vi "Teleop.vi"(10 "Match Info":T1={"Autonomous Elapsed Seconds"=0.0, "TeleOp Elapsed Seconds"=0.0, "Disabled Elapsed Seconds"=0.0, "Visited Autonomous"=FALSE, "Visited TeleOp"=FALSE, "Visited Disabled"=FALSE, "Autonomous Settings"={"Autonomous Style"=enum."Independent", "VI Refnum"=refnum}}, 11 "Call Context":T2) -> ()   [LabVIEW 2015]
doc: "This VI is called for each TeleOp packet received from the DS where the robot is not disabled. It is often used to read from the joysticks and update I/O or to update setpoints for timed control loops. It should complete and return within 20 milliseconds or it may miss DS packets."
uses:
  <vilib>/Rock Robotics/WPI/DriverStation/WPI_DriverStationDerivedRobotMode.ctl
  <vilib>/Rock Robotics/WPI/DriverStation/WPI_DriverStationMatch Info.ctl
  <vilib>/Rock Robotics/Network Tables/NT Read Boolean.vi
  <vilib>/Rock Robotics/Network Tables/NT Read Number.vi
  <vilib>/Rock Robotics/WPI/Utilities/WPI_GetSetVariantRefNum.vi
  Robot Global Data.vi
  <vilib>/Rock Robotics/Network Tables/SD Write Boolean.vi
  <vilib>/Rock Robotics/Network Tables/SD Write Number.vi
  navX Library v2/navX Library v2.lvlib
panel:
  in  "Speed":dbl
  out "Sample Slider 0":dbl(slide) scale=0.0..5.0
  out "Sample Boolean 1":bool
  out "Sample Boolean 0":bool
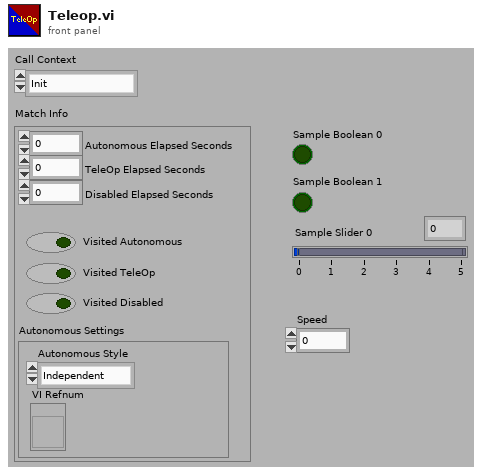
[diagram p1: front panel]
types:
  T1 = typedef "WPI_DriverStationMatch Info.ctl" = cluster{"Autonomous Elapsed Seconds":dbl, "TeleOp Elapsed Seconds":dbl, "Disabled Elapsed Seconds":dbl, "Visited Autonomous":bool, "Visited TeleOp":bool, "Visited Disabled":bool, "Autonomous Settings":cluster{"Autonomous Style":enum16{"Iterative", "Independent"}, "VI Refnum":refnum<vi>}}
  T2 = typedef "WPI_DriverStationDerivedRobotMode.ctl" = enum16{"Init", "Execute", "Stop"}
  T3 = typedef "navX Library v2.lvlib/Z900_navX_DeviceTypeDef.ctl" = cluster{"Interface":cluster{"Protocol":T4, "Update Rate (4Hz-60Hz)":u8, "navX Open TypeDef":variant}, "Notify Packet":refnum<notifier>, "Loop VI Refnum":refnum<vi>, "Ready to Close Occurrence Refnum":refnum<k4>}
  T4 = typedef "navX Library v2.lvlib/Z900_navX_ProtocolTypeDef.ctl" = enum16{"SERIAL", "I2C", "SPI"}
  T5 = cluster{"LinearAcceleration X":dbl, "LinearAcceleration Y":dbl, "LinearAcceleration Z":dbl}
  T6 = cluster{"Velocity X":dbl, "Velocity Y":dbl, "Velocity Z":dbl, "Displacement X":dbl, "Displacement Y":dbl, "Displacement Z":dbl}
  T7 = cluster{"Quat W":dbl, "Quat X":dbl, "Quat Y":dbl, "Quat Z":dbl}
  T8 = cluster{"Yaw":dbl, "Roll":dbl, "Pitch":dbl, "Heading":dbl, "Fused Heading":dbl}
  T9 = typedef "WPI_JoystickDevRef.ctl" = cluster{"Device":T10}
  T10 = typedef "WPI_JoystickDeviceEnum.ctl" = enum16{"USB 0", "USB 1", "USB 2", "USB 3", "USB 4", "USB 5"}
  T11 = cluster{"Axes[0]":dbl, "Axes[1]":dbl, "Axes[2]":dbl, "Axes[3]":dbl, "Axes[4]":dbl, "Axes[5]":dbl, "Axes[6]":dbl, "Axes[7]":dbl, "Axes[8]":dbl}
  T12 = cluster{"Buttons[0]":bool, "Buttons[1]":bool, "Buttons[2]":bool, "Buttons[3]":bool, "Buttons[4]":bool, "Buttons[5]":bool, "Buttons[6]":bool, "Buttons[7]":bool, "Buttons[8]":bool}
  T13 = typedef "WPI_EncoderDevRef.ctl" = cluster{"DevStatus":errorcluster, "EncoderIndex":T14, "CounterIndex":T15, "DistancePerCount":dbl, "Decoding Type":T16}
  T14 = typedef "FPGA_EncoderIdx.ctl" = enum8{"Enc 0", "Enc 1", "Enc 2", "Enc 3", "Enc 4", "Enc 5", "Enc 6", "Enc 7", "Invalid"}
  T15 = typedef "FPGA_CounterCtrSystemIndex.ctl" = enum8{"Ctr 0", "Ctr 1", "Ctr 2", "Ctr 3", "Ctr 4", "Ctr 5", "Ctr 6", "Ctr 7", "Invalid"}
  T16 = typedef "WPI_EncoderType.ctl" = enum16{"1x", "2x", "4x"}
  T17 = typedef "WPI_RobotDriveDevRef.ctl" = cluster{"DevStatus":errorcluster, "Motors[]":T18[], "Square Inputs":bool, "Max Output":dbl}
  T18 = typedef "WPI_MotorControlDeviceRef.ctl" = cluster{"DeviceStatus":errorcluster, "Type":T19, "PWM":cluster{"PWM Channel":T20, "DeadBand":T21}, "CAN":cluster{"Device Number":u8, "Control Mode":T22, "Semaphore":T23, "Max Vout":dbl, "TalonSRX Control Mode":T24}, "Invert":bool}
  T19 = typedef "WPI_MotorControlType.ctl" = enum16{"PWM", "CAN", "CANTalonSRX"}
  T20 = typedef "FPGA_DIOPWMChannel.ctl" = enum8{"PWM 0", "PWM 1", "PWM 2", "PWM 3", "PWM 4", "PWM 5", "PWM 6", "PWM 7", "PWM 8", "PWM 9", "PWM MXP 0", "PWM MXP 1", "PWM MXP 2", "PWM MXP 3", "PWM MXP 4", "PWM MXP 5", "PWM MXP 6", "PWM MXP 7", "PWM MXP 8", "PWM MXP 9", "Invalid"}
  T21 = typedef "WPI_PWMDeadband.ctl" = cluster{"Name":string, "maxPositivePwm":i32, "minPositivePwm":i32, "centerPwm":i32, "maxNegativePwm":i32, "minNegativePwm":i32, "angularRange":u16}
  T22 = typedef "WPI_CANJaguar_ControlMode.ctl" = enum8{"Percent VBus", "Current", "Speed", "Position", "Voltage"}
  T23 = typedef "Semaphore RefNum" = refnum<k1>
  T24 = typedef "WPI_CANTalonSRX_APIControlMode.ctl" = enum8{"Percent VBus", "Speed", "Position", "Slave", "Unchanged / Invalid", "Voltage Compensation", "Current", "Motion Profile"}
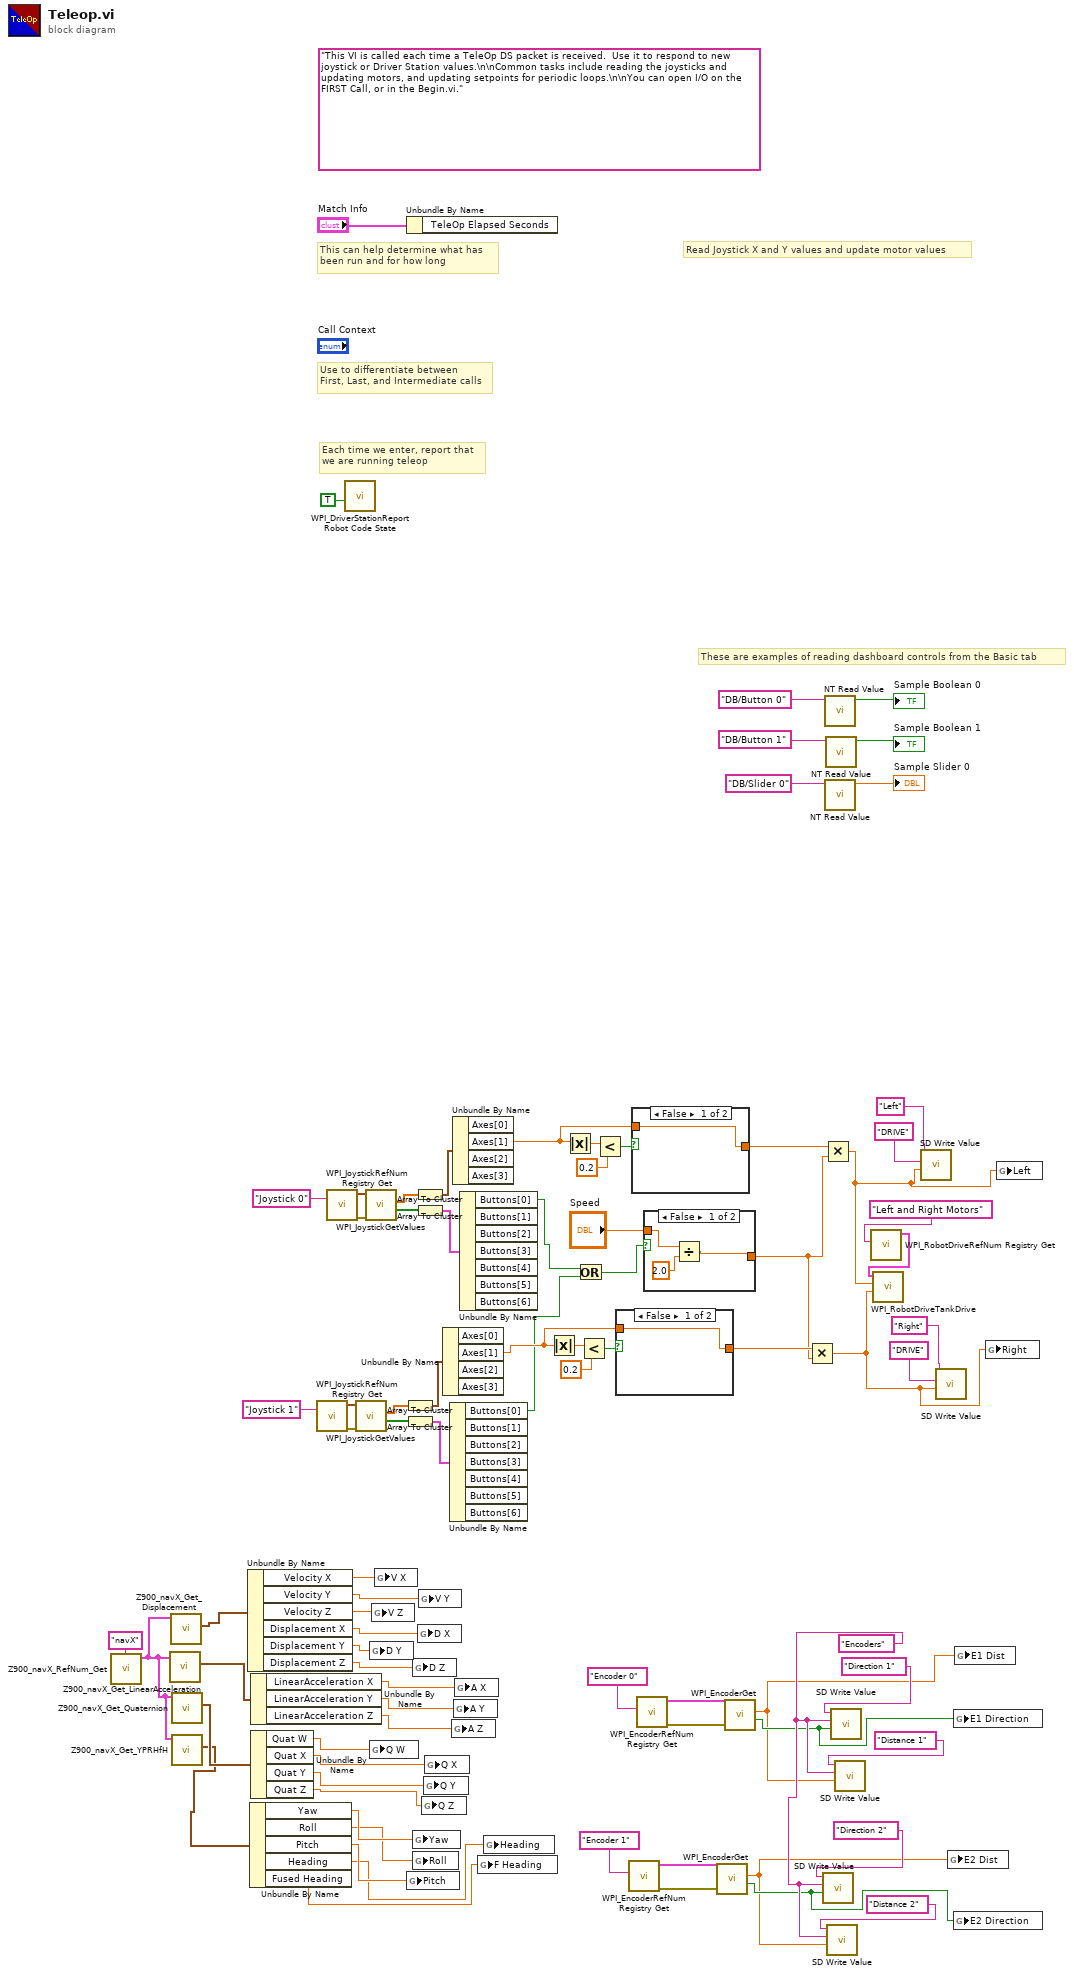
[diagram p0: block diagram]
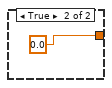
[diagram p3: hidden frame]
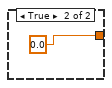
[diagram p4: hidden frame]
diagram:
  w33 = "Encoders"
  (unwired) "This VI is called each time a TeleOp DS packet is received.  Use it to respond to new joystick or Driver Station values.\n\nCommon tasks include reading the joysticks and updating motors, and updating setpoints for periodic loops.\n\nYou can open I/O on the FIRST Call, or in the Begin.vi."
  # "These are examples of reading dashboard controls from the Basic tab"
  # "Each time we enter, report that\nwe are running teleop"
  # "Use to differentiate between\nFirst, Last, and Intermediate calls"
  # "This can help determine what has\nbeen run and for how long"
  # "Read Joystick X and Y values and update motor values"
  n1 = call "Z900_navX_RefNum_Get.vi"("refnum name"="navX") -> ("navX Device"=w24:T3)  [unwired: 9 in, 1 out]
  n2 = call "Z900_navX_Get_LinearAcceleration.vi"("navX Device"=w24) -> ("Linear Acceleration"=w22:T5)  [unwired: 7 in, 3 out]
  n3 = call "Z900_navX_Get_Displacement.vi"("navX Device"=w24) -> ("Displacement"=w23:T6)  [unwired: 7 in, 3 out]
  n4 = call "Z900_navX_Get_Quaternion.vi"("navX Device"=w24) -> ("Quaternion"=w21:T7)  [unwired: 7 in, 3 out]
  n5 = call "Z900_navX_Get_YPRHfH.vi"("navX Device"=w24) -> ("YRPHfH"=w20:T8)  [unwired: 7 in, 3 out]
  n6 = Unbundle By Name(w23) -> ("Velocity X"=w18:dbl, "Velocity Y"=w17:dbl, "Velocity Z"=w16:dbl, "Displacement X"=w15:dbl, "Displacement Y"=w14:dbl, "Displacement Z"=w13:dbl)
  n7 = Unbundle By Name(w20) -> ("Yaw"=w6:dbl, "Roll"=w5:dbl, "Pitch"=w4:dbl, "Heading"=w2:dbl, "Fused Heading"=w1:dbl)
  n8 = Unbundle By Name(w22) -> ("LinearAcceleration X"=w12:dbl, "LinearAcceleration Y"=w11:dbl, "LinearAcceleration Z"=w10:dbl)
  n9 = Unbundle By Name(w21) -> ("Quat W"=w3:dbl, "Quat X"=w9:dbl, "Quat Y"=w8:dbl, "Quat Z"=w7:dbl)
  n10 = call <vilib>:"WPI_JoystickRefNum Registry Get.vi"("refnum name"="Joystick 1") -> ("error out"=w68:errorcluster, "JoystickDevRef"=w25:T9)  [unwired: 9 in]
  n11 = call <vilib>:"WPI_JoystickRefNum Registry Get.vi"("refnum name"="Joystick 0") -> ("error out"=w75:errorcluster, "JoystickDevRef"=w74:T9)  [unwired: 9 in]
  n12 = call <vilib>:"WPI_DriverStationReport Robot Code State.vi"("TeleOp"=TRUE ("Autonomous")) -> ()  [unwired: 10 in, 1 out]
  n13 = call <vilib>:"WPI_JoystickGetValues.vi"("error in (no error)"=w68, "JoystickDevRef"=w25) -> ("Buttons"=w66:bool[], "Axes"=w67:dbl[])  [unwired: 5 in, 3 out]
  n14 = call <vilib>:"WPI_JoystickGetValues.vi"("error in (no error)"=w75, "JoystickDevRef"=w74) -> ("Buttons"=w72:bool[], "Axes"=w73:dbl[])  [unwired: 5 in, 3 out]
  n15 = global write "Robot Global Data.vi" "D Y"(w14) -> ()
  n16 = global write "Robot Global Data.vi" "Q W"(w3) -> ()
  n17 = global write "Robot Global Data.vi" "V Z"(w16) -> ()
  n18 = global write "Robot Global Data.vi" "V X"(w18) -> ()
  n19 = Array To Cluster(array=w67) -> (cluster=w65:T11)
  n20 = Array To Cluster(array=w66) -> (cluster=w64:T12)
  n21 = Unbundle By Name("Match Info") -> ()  [unwired: 1 out]
  n22 = global write "Robot Global Data.vi" "Pitch"(w4) -> ()
  n23 = global write "Robot Global Data.vi" "D Z"(w13) -> ()
  n24 = global write "Robot Global Data.vi" "Yaw"(w6) -> ()
  n25 = global write "Robot Global Data.vi" "Roll"(w5) -> ()
  n26 = Array To Cluster(array=w73) -> (cluster=w71:T11)
  n27 = Array To Cluster(array=w72) -> (cluster=w70:T12)
  n28 = global write "Robot Global Data.vi" "D X"(w15) -> ()
  n29 = global write "Robot Global Data.vi" "V Y"(w17) -> ()
  n30 = global write "Robot Global Data.vi" "Q Z"(w7) -> ()
  n31 = global write "Robot Global Data.vi" "Q Y"(w8) -> ()
  n32 = global write "Robot Global Data.vi" "Q X"(w9) -> ()
  n33 = Unbundle By Name(w65) -> ("Axes[1]"=w54:dbl)  [unwired: 3 out]
  n34 = Unbundle By Name(w64) -> ("Buttons[0]"=w45:bool)  [unwired: 6 out]
  n35 = global write "Robot Global Data.vi" "A Z"(w10) -> ()
  n36 = Unbundle By Name(w71) -> ("Axes[1]"=w59:dbl)  [unwired: 3 out]
  n37 = global write "Robot Global Data.vi" "A Y"(w11) -> ()
  n38 = global write "Robot Global Data.vi" "A X"(w12) -> ()
  n39 = Unbundle By Name(w70) -> ("Buttons[0]"=w46:bool)  [unwired: 6 out]
  n40 = global write "Robot Global Data.vi" "F Heading"(w1) -> ()
  n41 = global write "Robot Global Data.vi" "Heading"(w2) -> ()
  n42 = Absolute Value(x=w54) -> (abs(x)=w58:dbl)
  n43 = Absolute Value(x=w59) -> (abs(x)=w63:dbl)
  n44 = Or(x=w46, y=w45) -> (x .or. y?=w44:bool)
  n45 = Less?(x=w58, y=0.2) -> (x < y?=w56:bool)
  n46 = Less?(x=w63, y=0.2) -> (x < y?=w61:bool)
  n47 = case shown="False" w56 {
    tunnel: [w85 0.0] -> w55
    tunnel: w54 -> [w85 _]
    frame False {
    }
    frame True {
    }
  }
  n48 = call <vilib>:"WPI_EncoderRefNum Registry Get.vi"("refnum name"="Encoder 1") -> ("error out"=w37:errorcluster, "EncoderDevRef"=w36:T13)  [unwired: 9 in]
  n49 = case shown="False" w61 {
    tunnel: [w87 0.0] -> w60
    tunnel: w59 -> [w87 _]
    frame False {
    }
    frame True {
    }
  }
  n50 = call <vilib>:"WPI_EncoderRefNum Registry Get.vi"("refnum name"="Encoder 0") -> ("error out"=w42:errorcluster, "EncoderDevRef"=w41:T13)  [unwired: 9 in]
  n51 = case shown="False" w44 {
    tunnel: [w90 w92] -> w53
    tunnel: "Speed" -> [w91 w92]
    frame False {
      n52 = Divide(x=w91, y=2.0) -> (x/y=w90:dbl)
    }
    frame True {
    }
  }
  n53 = call <vilib>:"WPI_EncoderGet.vi"("error in (no error)"=w37, "EncoderDevRef"=w36) -> ("Direction"=w31:bool, "Distance"=w29:dbl)  [unwired: 4 in, 4 out]
  n54 = call <vilib>:"WPI_EncoderGet.vi"("error in (no error)"=w42, "EncoderDevRef"=w41) -> ("Direction"=w32:bool, "Distance"=w30:dbl)  [unwired: 4 in, 4 out]
  n55 = Multiply(x=w55, y=w53) -> (x*y=w26:dbl)
  n56 = Multiply(x=w60, y=w53) -> (x*y=w27:dbl)
  n57 = call-poly <vilib>:"SD Write Value.vi"("Boolean"=w31, "Table Prefix"=w33, "Name"="Direction 2") -> ()  [unwired: 7 in, 2 out]
  n58 = call-poly <vilib>:"NT Read Value.vi"("Name"="DB/Button 0" ("refnum name")) -> ("Boolean"=→"Sample Boolean 0":bool)  [unwired: 9 in, 1 out]
  n59 = call-poly <vilib>:"NT Read Value.vi"("Name"="DB/Slider 0" ("refnum name")) -> ("Numeric"=→"Sample Slider 0":dbl)  [unwired: 9 in, 1 out]
  n60 = call-poly <vilib>:"NT Read Value.vi"("Name"="DB/Button 1" ("refnum name")) -> ("Boolean"=→"Sample Boolean 1":bool)  [unwired: 9 in, 1 out]
  n61 = call-poly <vilib>:"SD Write Value.vi"("Numeric"=w29, "Table Prefix"=w33, "Name"="Distance 2") -> ()  [unwired: 7 in, 2 out]
  n62 = call-poly <vilib>:"SD Write Value.vi"("Boolean"=w32, "Table Prefix"=w33, "Name"="Direction 1") -> ()  [unwired: 7 in, 2 out]
  n63 = call-poly <vilib>:"SD Write Value.vi"("Numeric"=w30, "Table Prefix"=w33, "Name"="Distance 1") -> ()  [unwired: 7 in, 2 out]
  n64 = call <vilib>:"WPI_RobotDriveRefNum Registry Get.vi"("refnum name"="Left and Right Motors") -> ("RobotDriveDevRef"=w52:T17)  [unwired: 9 in, 1 out]
  n65 = call <vilib>:"WPI_RobotDriveTankDrive.vi"("Right axis value"=w26, "Left axis value"=w27, "RobotDriveDevRef"=w52) -> ()  [unwired: 6 in, 3 out]
  n66 = call-poly <vilib>:"SD Write Value.vi"("Numeric"=w27, "Table Prefix"="DRIVE", "Name"="Left") -> ()  [unwired: 7 in, 2 out]
  n67 = call-poly <vilib>:"SD Write Value.vi"("Numeric"=w26, "Table Prefix"="DRIVE", "Name"="Right") -> ()  [unwired: 7 in, 2 out]
  n68 = global write "Robot Global Data.vi" "E2 Dist"(w29) -> ()
  n69 = global write "Robot Global Data.vi" "E1 Direction"(w32) -> ()
  n70 = global write "Robot Global Data.vi" "E2 Direction"(w31) -> ()
  n71 = global write "Robot Global Data.vi" "E1 Dist"(w30) -> ()
  n72 = global write "Robot Global Data.vi" "Right"(w26) -> ()
  n73 = global write "Robot Global Data.vi" "Left"(w27) -> ()
